vi "提取日志报警参数入列队 (子VI).vi"(10 "枚举":enum16{"CODMn", "氨氮", "总磷", "总氮", "数采仪"}(ring), 11 "队列输入":refnum<queue>) -> ()   [LabVIEW 2016]
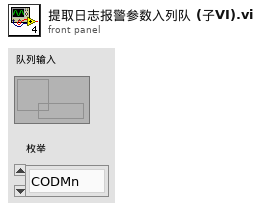
[diagram p1: front panel]
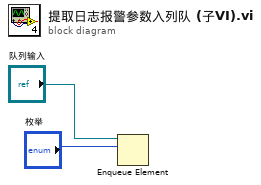
[diagram p0: block diagram]
diagram:
  n1 = Enqueue Element(queue="队列输入", element="枚举") -> ()  [unwired: 2 in, 3 out]
